vi "test_agv.vi"() -> ()   [LabVIEW 2018]
panel:
  out "error":bool
  out "agv data out":T1
  out "speed chart":T2(graph)
  in  "buf mode":bool=TRUE
  in  "agv_cmd":cluster{"v_linear":dbl, "v_angular":dbl}={"v_linear"=0.0, "v_angular"=0.2} {"v_angular" min=-0.5 max=0.5 scale=-0.5..0.5; "v_linear" min=-0.5 max=0.5 scale=-0.5..0.5}
  in  "정지":bool
  in  "AGV_Port":refnum<visa-resource-name>="COM5"
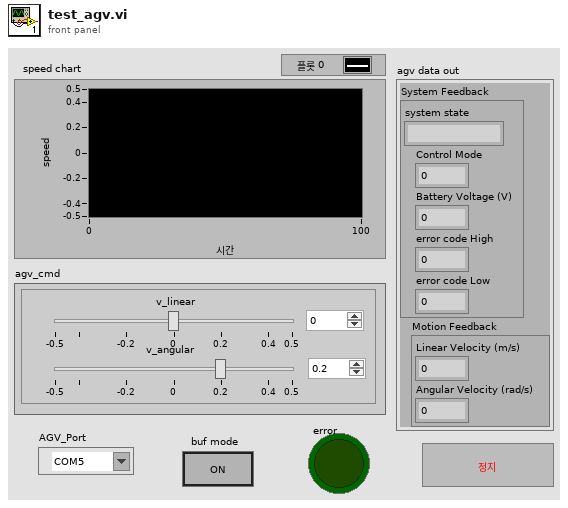
[diagram p1: front panel]
types:
  T1 = cluster{"System Feedback":cluster{"system state":string, "Control Mode":u8, "Battery Voltage (V)":dbl, "error code High":u8, "error code Low":u8}, "Motion Feedback":cluster{"Linear Velocity (m/s)":dbl, "Angular Velocity (rad/s)":dbl}}
  T2 = cluster{"linear_vel out":dbl, "angle_vel out":dbl}
  T3 = cluster{"Port":refnum<visa-resource-name>, "speed limits":cluster{"limit_linear-v":dbl, "limit_angular-v":dbl}}
  T4 = cluster{"System Feedback":cluster{"system state":string, "Control Mode":u8, "Battery Voltage":dbl, "error code High":u8, "error code Low":u8}, "Motion Feedback":cluster{"Linear Velocity (m/s)":dbl, "Angular Velocity (rad/s)":dbl}}
  T5 = cluster{"Linear Velocity":dbl, "Angular Velocity":dbl}
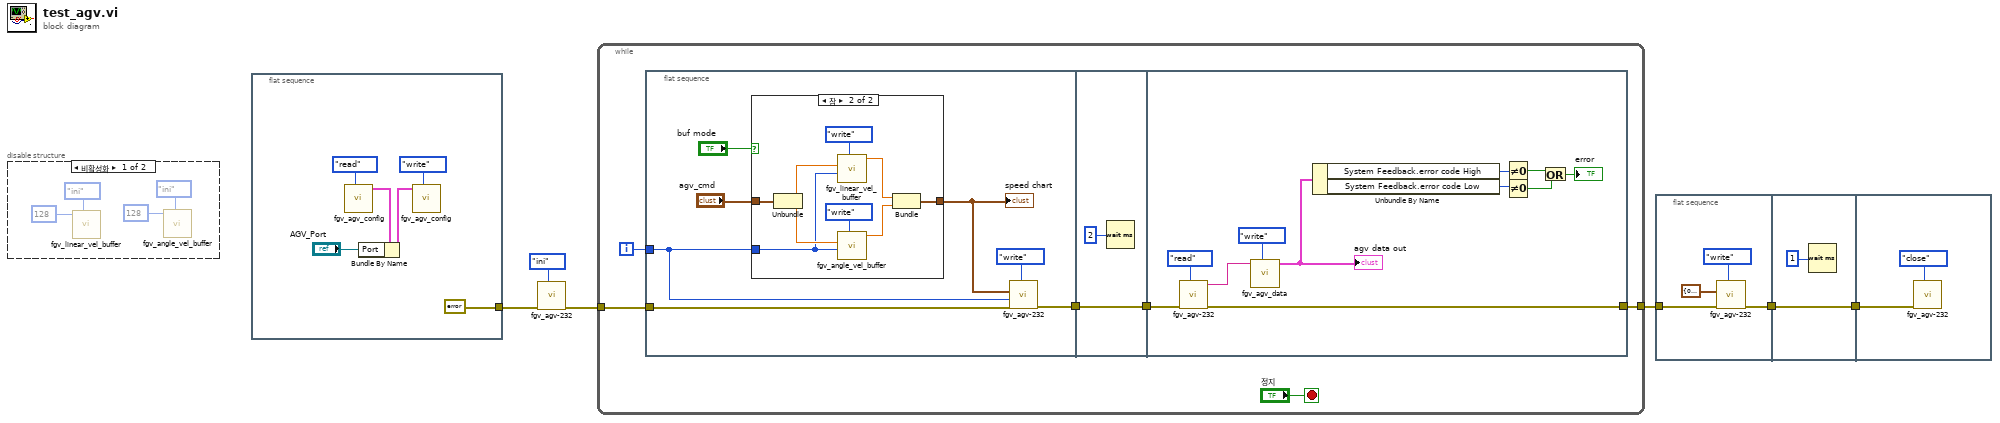
[diagram p0: block diagram]
diagram:
  n1 = disable-structure shown="비활성화" {
    frame Disabled {
      n2 = call "fgv_linear_vel_buffer.vi"("agv_cmd_angle"=enum16{"ini", "write", "read"}."ini", "dim size"=128) -> ()  [unwired: 9 in, 1 out]
      n3 = call "fgv_angle_vel_buffer.vi"("agv_cmd_angle"=enum16{"ini", "write", "read"}."ini", "dim size"=128) -> ()  [unwired: 9 in, 1 out]
    }
    frame Enabled {
    }
  }
  n4 = flat-sequence {
    tunnel: [errorcluster {"status"=FALSE, "code"=0, "source"=""} ("error in")] -> w3
    frame #0 {
      n5 = call "fgv_agv_config.vi"("cmd"=enum16{"read", "write"}."read") -> ("AGV cfg out"=w13:T3)  [unwired: 10 in]
      n6 = Bundle By Name(cluster=w13, "Port"="AGV_Port") -> (w12:T3)
      n7 = call "fgv_agv_config.vi"("cmd"=enum16{"read", "write"}."write", "AGV cfg"=w12) -> ()  [unwired: 9 in, 1 out]
    }
  }
  n8 = call "fgv_agv-232.vi"("cmd"=enum16{"ini", "write", "read", "close"}."ini", "error in"=w3) -> ("error out"=w5:errorcluster)  [unwired: 7 in, 2 out]
  n9 = while {
    tunnel: w5 -> [w20]
    tunnel: [w17] -> w4
    i -> [w21]
    stop <- "정지" stop-if-true
    n10 = flat-sequence {
      tunnel: w21 -> [w25]
      tunnel: w20 -> [w28]
      tunnel: [w27] -> w18
      tunnel: [w41] -> w19
      tunnel: w18 -> [w41]
      tunnel: w19 -> [w51]
      tunnel: [w50] -> w17
      frame #0 {
        n11 = case shown="참" "buf mode" {
          tunnel: [w30 w39] -> w23
          tunnel: w25 -> [_ w31]
          tunnel: "agv_cmd" -> [w30 w36]
          frame False {
          }
          frame True {
            n12 = Unbundle(w36) -> ("v_linear"=w35:dbl, "v_angular"=w34:dbl)
            n13 = call "fgv_linear_vel_buffer.vi"("agv_cmd_angle"=enum16{"ini", "write", "read"}."write", "index"=w31, "linear_vel in"=w35) -> ("linear_vel out"=w37:dbl)  [unwired: 8 in]
            n14 = call "fgv_angle_vel_buffer.vi"("agv_cmd_angle"=enum16{"ini", "write", "read"}."write", "index"=w31, "angle_vel in"=w34) -> ("angle_vel out"=w38:dbl)  [unwired: 8 in]
            n15 = Bundle("linear_vel out"=w37, "angle_vel out"=w38) -> (w39:T2)  [unwired: 1 in]
          }
        }
        "speed chart" <- w23
        n16 = call "fgv_agv-232.vi"("cmd"=enum16{"ini", "write", "read", "close"}."write", "error in"=w28, "Frame ID"=w25, "control-val"=w23) -> ("error out"=w27:errorcluster)  [unwired: 5 in, 2 out]
      }
      frame #1 {
        n17 = Wait (ms)(milliseconds to wait=u32 2) -> ()  [unwired: 1 out]
      }
      frame #2 {
        n18 = call "fgv_agv-232.vi"("cmd"=enum16{"ini", "write", "read", "close"}."read", "error in"=w51) -> ("error out"=w50:errorcluster, "read data"=w48:string)  [unwired: 7 in, 1 out]
        n19 = call "fgv_agv_data.vi"("cmd"=enum16{"write", "read"}."write", "raw data"=w48) -> ("agv data out"=w47:T4)  [unwired: 9 in]
        "agv data out" <- w47
        n20 = Unbundle By Name(w47) -> ("System Feedback.error code High"=w46:u8, "System Feedback.error code Low"=w45:u8)
        n21 = Not Equal To 0?(x=w46) -> (x != 0?=w44:bool)
        n22 = Not Equal To 0?(x=w45) -> (x != 0?=w42:bool)
        n23 = Or(x=w44, y=w42) -> (x .or. y?=→"error":bool)
      }
    }
  }
  n24 = flat-sequence {
    tunnel: w4 -> [w54]
    tunnel: [w53] -> w1
    tunnel: [w58] -> w2
    tunnel: w1 -> [w58]
    tunnel: w2 -> [w59]
    frame #0 {
      n25 = call "fgv_agv-232.vi"("cmd"=enum16{"ini", "write", "read", "close"}."write", "error in"=w54, "control-val"=T5 {"Linear Velocity"=0.0, "Angular Velocity"=0.0}) -> ("error out"=w53:errorcluster)  [unwired: 6 in, 2 out]
    }
    frame #1 {
      n26 = Wait (ms)(milliseconds to wait=u32 1) -> ()  [unwired: 1 out]
    }
    frame #2 {
      n27 = call "fgv_agv-232.vi"("cmd"=enum16{"ini", "write", "read", "close"}."close", "error in"=w59) -> ()  [unwired: 7 in, 3 out]
    }
  }
